vi "Main Loop.vi"(8 "error in (no error)":errorcluster, 10 "Chart Notifier":refnum<notifier>, 11 "Message Queues":T1) -> (0 "error out":errorcluster)   [LabVIEW 2018, in "Centrifuge Module.lvlib" / "Centrifuge Module Engine.lvlib"]
uses:
  Centrifuge Module Engine.lvlib
  All Message Queues.ctl
  support/Message Queue/Message Cluster.ctl
  State Cluster.ctl
  State Enum.ctl
  Centrifuge Module Settings Cluster.ctl
  EPOS4/Controls/Device Selection.ctl
  EPOS4/Controls/EPOS Communication Settings.ctl
  Centrifuge Module Display.ctl
  <vilib>/Platform/TimedLoop/XDataNode/timing_clust.ctl
  <vilib>/Platform/TimedLoop/XDataNode/nitl_modes.ctl
  <vilib>/Platform/TimedLoop/XDataNode/wakeup.ctl
  Tag VIs/Tag FGV Operation Enum.ctl
  support/Message Queue/Enqueue Message (Single).vi
  <vilib>/Platform/TimedLoop/XDataNode/XDataNode.xnode
  support/Message Queue/Message Queue.lvlib
  <vilib>/Platform/TimedLoop/XDataNode/XDNodeRunTimeDep.lvlib
  Centrifuge Module.lvlib
  Shared Variables/Dynamic Shared Variables.lvlib
  support/Support Library.lvlib
  EPOS4/EPOS4.lvlib
panel:
  out "Period (s)":dbl format="%_4g"
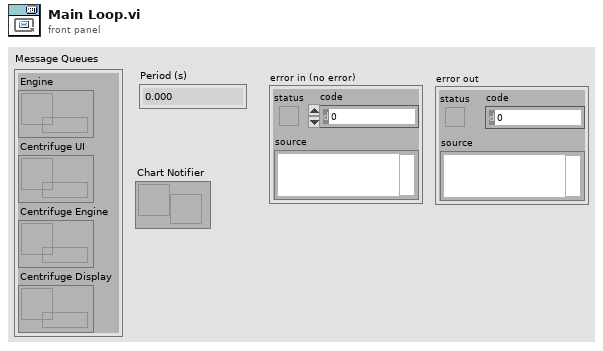
[diagram p1: front panel]
types:
  T1 = typedef "Centrifuge Module.lvlib/All Message Queues.ctl" = cluster{"Engine":refnum<queue>, "Centrifuge UI":refnum<queue>, "Centrifuge Engine":refnum<queue>, "Centrifuge Display":refnum<queue>}
  T2 = typedef "Centrifuge Module.lvlib/Centrifuge Module Display.ctl" = cluster{"Centrifuge On?":enum16{"Off", "On", "Not Initialized"}, "Cycle Period":dbl, "Current Centrifuge Speed":dbl, "Output":T3}
  T3 = typedef "Device Selection.ctl" = enum16{"Default", "EPOS4"}
  T4 = typedef "XDNodeRunTimeDep.lvlib/timing_clust.ctl" = cluster{"Expected End [f-1]":u64, "Actual End [f-1]":u64, "Finished Late? [f-1]":bool, "Expected End [i-1]":u64, "Actual End [i-1]":u64, "Finished Late? [i-1]":bool, "Expected Start [i]":u64, "Actual Start [i]":u64, "Expected Start [f]":u64, "Actual Start [f]":u64, "Source Name":string, "Structure Name":string, "Period":i64, "Deadline":i64, "Offset":i64, "Start":i64, "Priority":i32, "Timeout":i32, "Mode":T5, "Wakeup Reason":T6, "Error":errorcluster, "Source Type":string, "Secondary Source Type":string, "Global End Time":u64, "Global Start Time":u64, "Frame Duration":u64, "Iteration Duration":u64, "Assigned CPU":i32, "I/O Scan Engine Mode":u32}
  T5 = typedef "XDNodeRunTimeDep.lvlib/nitl_modes.ctl" = enum32{"No Change", "Process missed periods, maintain original phase", "Discard missed periods, maintain original phase", "Process missed periods, ignore original phase", "Discard missed periods, ignore original phase"}
  T6 = typedef "XDNodeRunTimeDep.lvlib/wakeup.ctl" = enum32{"Normal", "Aborted", "Asynchronous wakeup", "Timing source error", "Timed loop error", "Timeout"}
  T7 = cluster{"enable? (F)":bool, "name":string, "alarm on":bool, "priority":u32, "ack type":enum16{"Auto", "User", "None", "Each Occurrence"}, "area":string, "description":string, "log? (T)":bool}
  T8 = typedef "Tag FGV Operation Enum.ctl" = enum16{"Init", "Set Notification Queue", "Create Tag", "Commit", "Write Tag (Numeric)", "Write Tag (Boolean)", "Read All Tags", "Read One Tag", "Delete Tag Category", "Set Alarm Parameters (Numeric)", "Set Alarm Parameters (Boolean)", "Enable All Alarms", "Disable All Alarms", "Delete All Tags", "Read Alarms", "Ack Alarm", "Read Alarm Parameters (Numeric)", "Read Alarm Parameters (Boolean)"}
  T9 = enum32{"u32BitField", "bool", "double", "string", "int8", "uint8", "int16", "uint16", "int32", "uint32", "int64", "uint64", "single", "double waveform", "int16 waveform", "array of boolean", "array of int8", "array of uint8", "array of int16", "array of uint16", "array of int32", "array of uint32", "array of int64", "array of uint64", "array of single", "array of double", "array of double waveform", "array of int16 waveform", "array of string", "variant", "timestamp", "fixed point", "custom"}
  T10 = typedef "Centrifuge Module.lvlib/Centrifuge Module Engine.lvlib/State Enum.ctl" = enum16{"Measuring", "Idle", "Paused"}
  T11 = typedef "Centrifuge Module.lvlib/Centrifuge Module Engine.lvlib/State Cluster.ctl" = cluster{"State":T10, "Start Time":timestamp, "Configuration":T12, "Current Time":timestamp, "First Iteration":bool, "Data":cluster{"Centrifuge Speed":dbl}, "Process Name":string, "Centrifuge On?":enum16{"Off", "On", "Not Initialized"}, "Output Error":bool, "Log Started":bool}
  T12 = typedef "Centrifuge Module.lvlib/Centrifuge Module Settings Cluster.ctl" = cluster{"Cycle Period":dbl, "Manual Entry":dbl, "Output Device":T3, "EPOS4 Settings":T13}
  T13 = typedef "EPOS4.lvlib/EPOS Communication Settings.ctl" = cluster{"VISA resource name":refnum<visa-resource-name>, "axis":cluster{"keyHandle":u32, "nodeId":u16}, "Simulated?":bool}
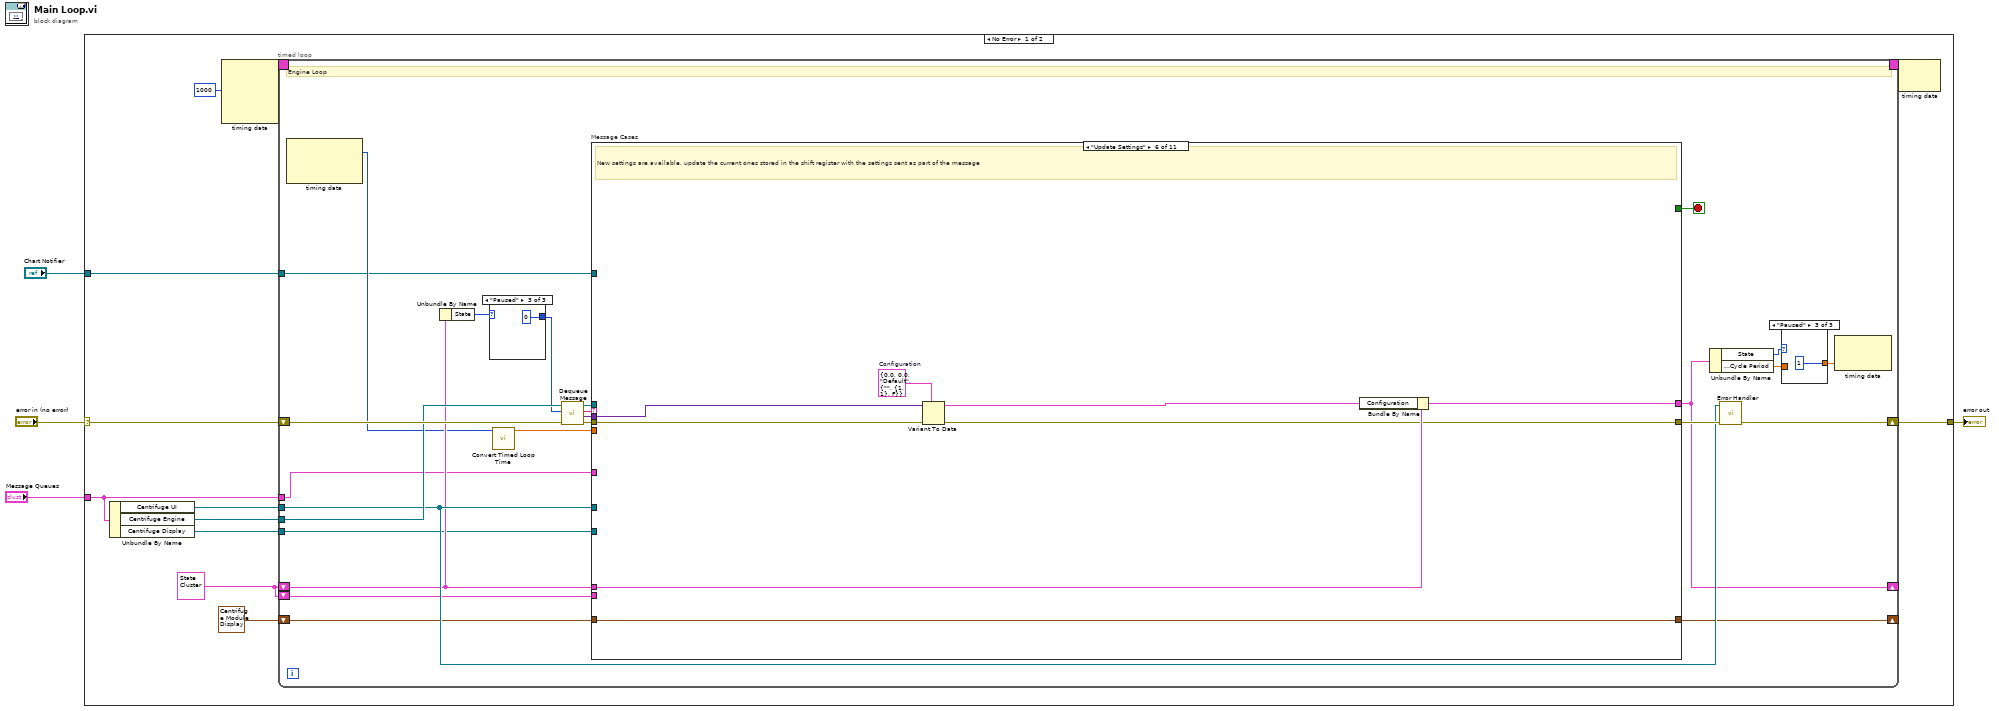
[diagram p0: block diagram]
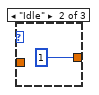
[diagram p3: hidden frame]
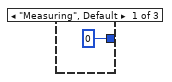
[diagram p4: hidden frame]
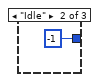
[diagram p5: hidden frame]
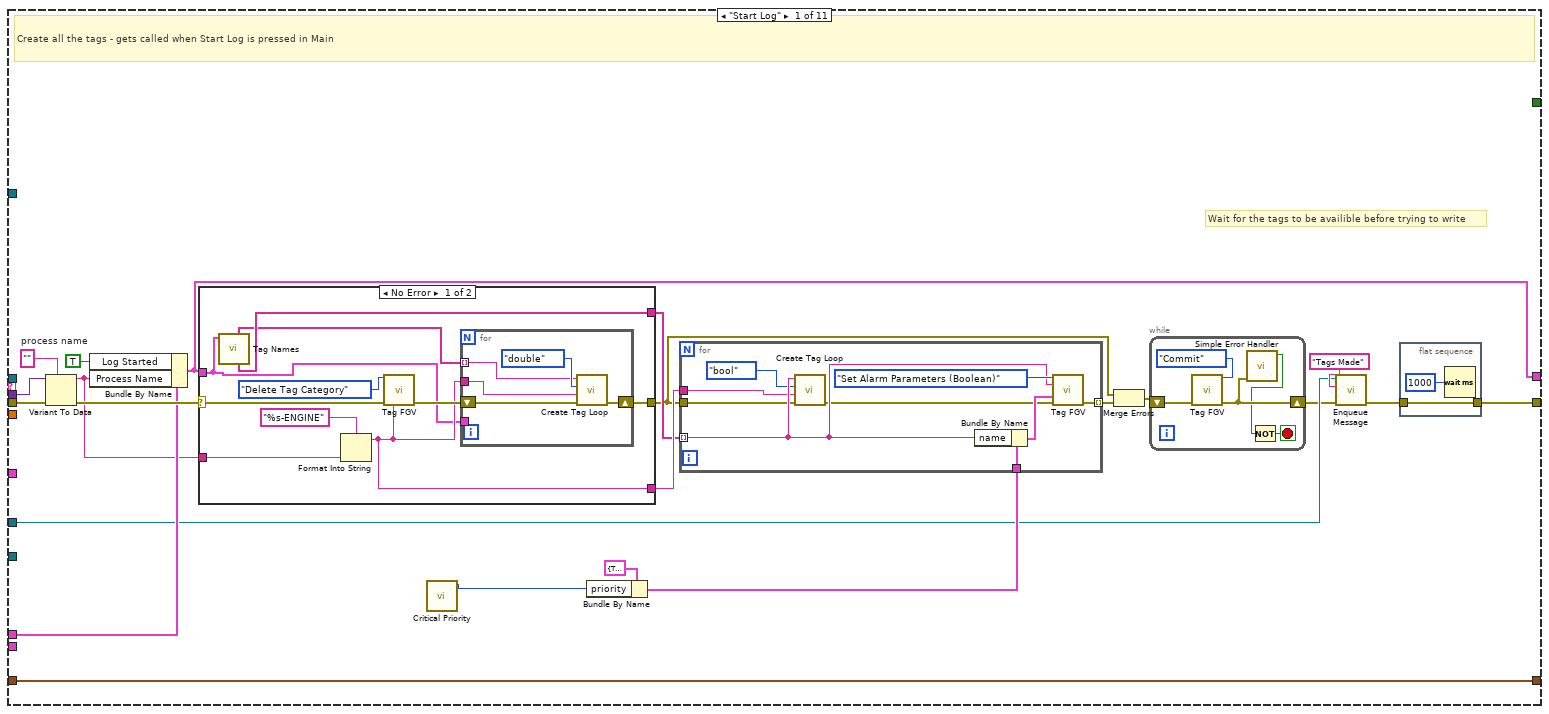
[diagram p6: hidden frame]
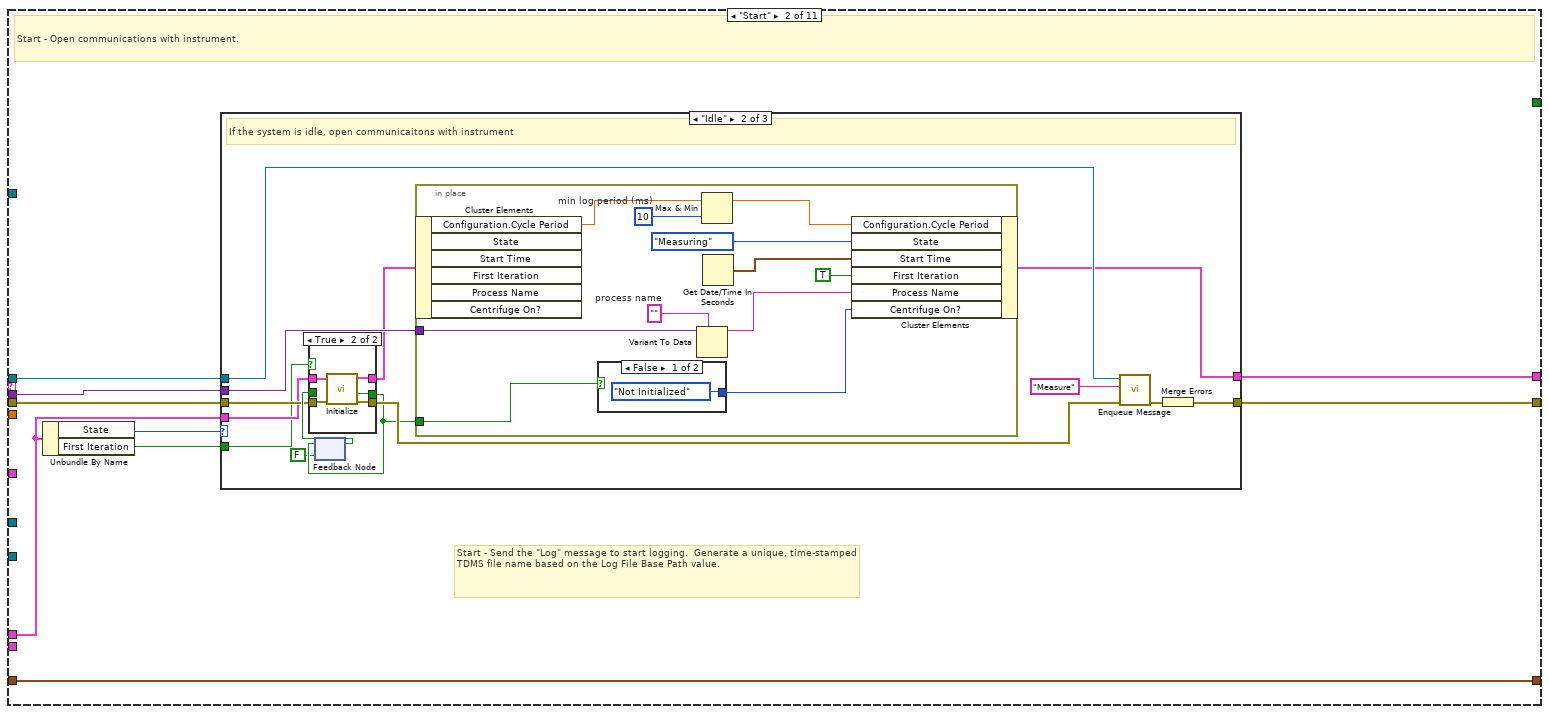
[diagram p8: hidden frame]
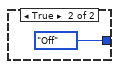
[diagram p10: hidden frame]
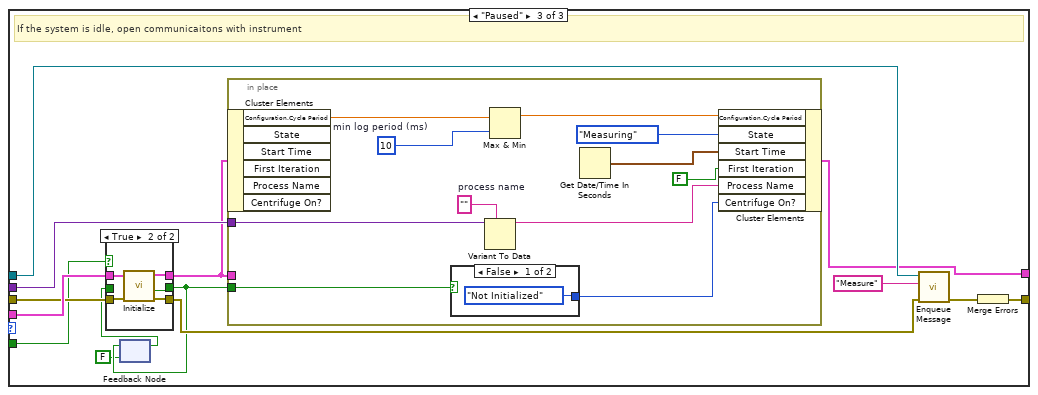
[diagram p12: hidden frame]
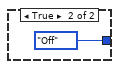
[diagram p13: hidden frame]
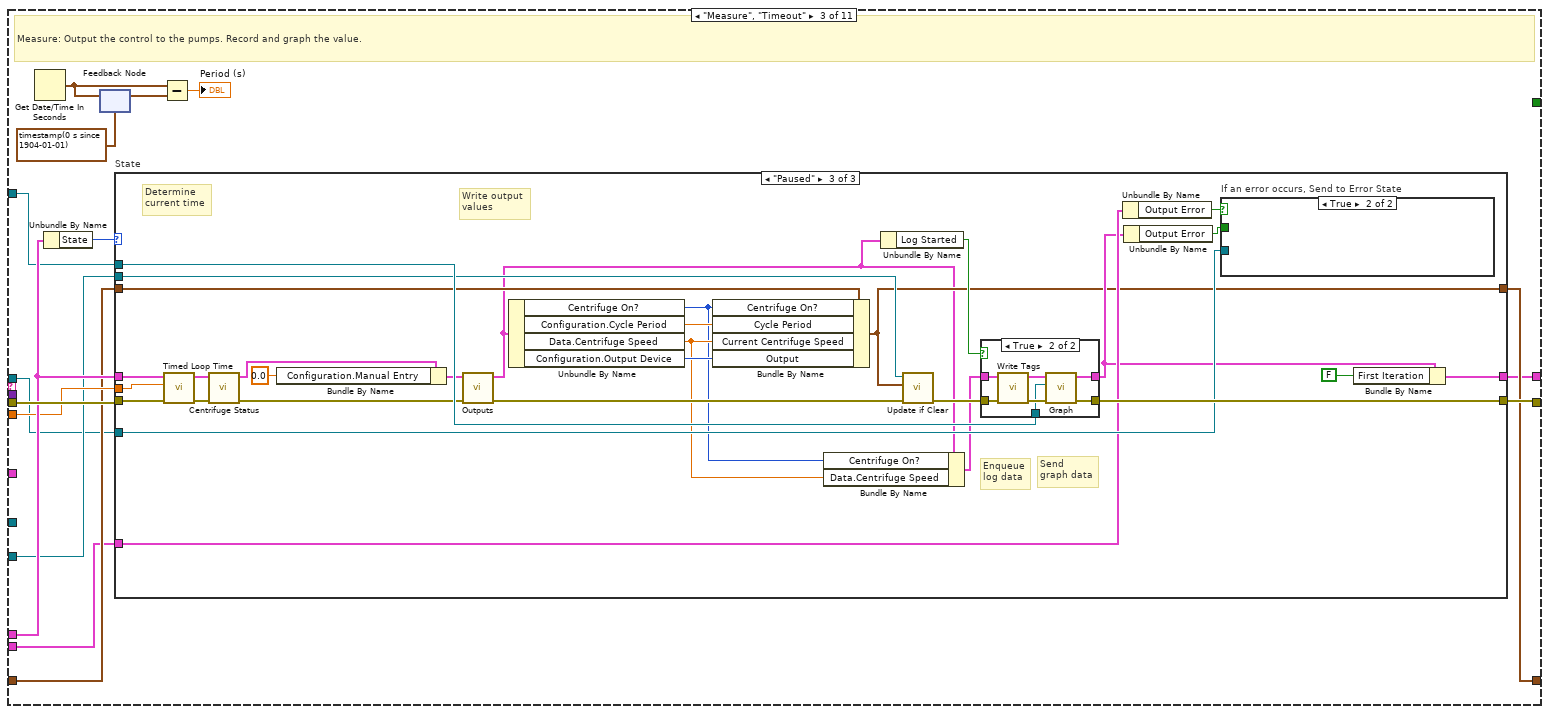
[diagram p15: hidden frame]
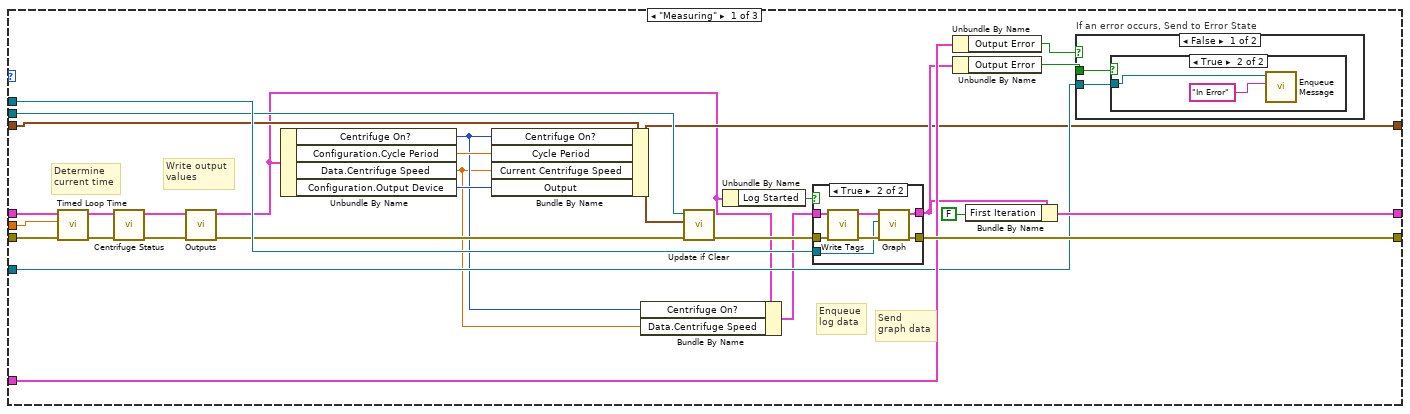
[diagram p16: hidden frame]
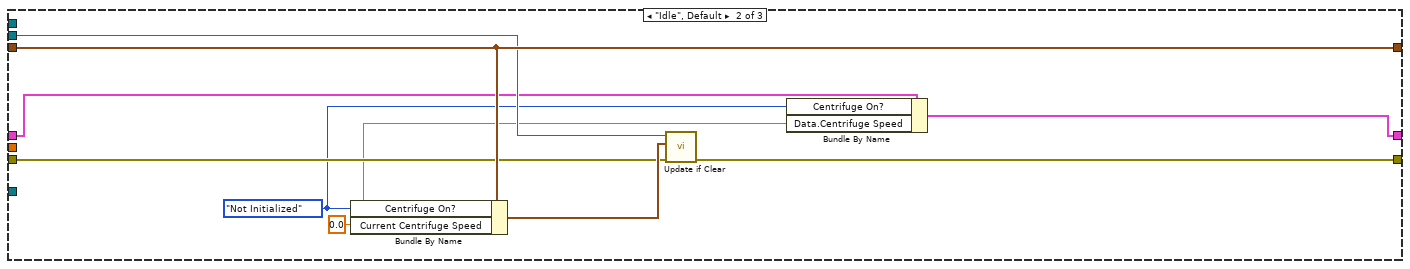
[diagram p20: hidden frame]
diagram:
  n1 = case shown="No Error" "error in (no error)" {
    selector: "error in (no error)" -> [w15 w414]
    tunnel: "Message Queues" -> [w11 _]
    tunnel: [w16 w414] -> w3
    tunnel: "Chart Notifier" -> [w9 _]
    frame No Error {
      w6 = T11 {"State"=enum."Idle", "Start Time"=timestamp(0 s since 1904-01-01), "Configuration"={"Cycle Period"=0.0, "Manual Entry"=0.0, "Output Device"=enum."Default", "EPOS4 Settings"={"VISA resource name"="", "axis"={"keyHandle"=1, "nodeId"=1}, "Simulated?"=FALSE}}, "Current Time"=timestamp(0 s since 1904-01-01), "First Iteration"=FALSE, "Data"={"Centrifuge Speed"=0.0}, "Process Name"="", "Centrifuge On?"=enum."Off", "Output Error"=FALSE, "Log Started"=FALSE}
      n2 = Unbundle By Name(w11) -> ("Centrifuge UI"=w14:refnum<queue>, "Centrifuge Engine"=w10:refnum<queue>, "Centrifuge Display"=w8:refnum<queue>)
      n3 = node-c288(i64 1000 ("Period")) -> (w13:T4)  [unwired: 3 in]
      n4 = timed-loop {
        tunnel: w10 -> [w35]
        shift-right: [w17] -> _
        shift-left: w6 -> [w31]
        shift-right: [w33] -> w16
        shift-left: w15 -> [w40]
        tunnel: w14 -> [w32]
        timing: w13 -> [_]
        timing-out: [_] -> w12
        tunnel: w11 -> [w23]
        tunnel: w9 -> [w22]
        tunnel: w8 -> [w21]
        shift-right: [w20] -> _
        shift-left: T2 {"Centrifuge On?"=enum."Off", "Cycle Period"=500.0, "Current Centrifuge Speed"=0.0, "Output"=enum."Default"} ("PM Display") -> [w19]
        shift-left: w6 -> [w18]
        stop <- w41 stop-if-true
        # "Engine Loop"
        n5 = node-c288() -> (w25:i64)  [unwired: 1 in, 2 out]
        n6 = Unbundle By Name(w31) -> ("State"=w30:T10)
        n7 = case shown="\"Paused\"" w30 {
          tunnel: [0 ("timeout in ms (-1)") -1 ("timeout in ms (-1)") 0 ("timeout in ms (-1)")] -> w29
          frame "Measuring", Default {
          }
          frame "Idle" {
          }
          frame "Paused" {
          }
        }
        n8 = call "Convert Timed Loop Time.vi"("Actual Start [i]"=w25) -> ("ET since start (s)"=w24:dbl)  [unwired: 10 in]
        n9 = call "Dequeue Message.vi"("error in (no error)"=w40, "timeout in ms (-1)"=w29, "Message Queue"=w35) -> ("error out"=w39:errorcluster, "Message Data"=w37:variant, "Message"=w38:string, "dup Message Queue"=w36:refnum<queue>)  [unwired: 5 in]
        n10 = case "Message Cases" shown="\"Update Settings\"" w38 {
          selector: w38 -> [_ _ _ _ _ _ _ _ _ _ w403]
          tunnel: w36 -> [_ w114 w191 _ _ _ w357 _ w373 _ _]
          tunnel: w39 -> [w58 w113 w201 w302 w328 w351 w360 w367 w383 w401 _]
          tunnel: [w54 w115 w202 w297 w324 w347 w362 w366 w378 w400 w402] -> w34
          tunnel: w31 -> [w64 w110 w200 w304 w329 w348 w353 w364 w382 w398 w408]
          tunnel: [w60 w107 w189 w303 w331 w346 w353 w364 w379 w396 w408] -> w17
          tunnel: [_ _ _ _ _ _ TRUE _ _ _ _] -> w41
          tunnel: w37 -> [w73 w111 _ _ _ w352 _ _ _ _ _]
          tunnel: w32 -> [w61 _ _ w306 _ _ w361 _ _ _ _]
          tunnel: w24 -> [_ _ w199 _ _ _ _ _ _ _ _]
          tunnel: w23 -> [_ _ _ _ _ _ _ _ _ _ _]
          tunnel: w22 -> [_ _ w195 _ _ _ _ _ _ _ _]
          tunnel: w21 -> [_ _ w194 w300 w326 _ _ _ w372 _ _]
          tunnel: w19 -> [w74 w109 w193 w299 w325 w349 w354 w365 w376 w399 w409]
          tunnel: [w74 w109 w192 w299 w325 w349 w354 w365 w371 w399 w409] -> w20
          tunnel: w18 -> [_ _ w190 _ _ _ _ _ _ _ _]
          frame "Start Log" {
            w72 = ""  # process name
            # "Wait for the tags to be availible before trying to write"
            # "Create all the tags - gets called when Start Log is pressed in Main"
            n11 = Variant To Data(error in=w58, type=w72, Variant=w73) -> (data=w59:string, error out=w71:errorcluster)
            n12 = Bundle By Name(cluster=w64, "Log Started"=TRUE, "Process Name"=w59) -> (w60:T11)
            n13 = case shown="No Error" w71 {
              selector: w71 -> [w97 w106]
              tunnel: [w100 w106] -> w53
              tunnel: [w95 _] -> w67
              tunnel: [w94 _] -> w66
              tunnel: w60 -> [w91 _]
              tunnel: w59 -> [w93 _]
              frame No Error {
                n14 = call "Tag Names.vi"("State In"=w91) -> ("All Boolean Tags"=w94:string[], "All  Numeric Tags"=w92:string[])  [unwired: 8 in, 1 out]
                n15 = Format Into String(format string="%s-ENGINE", w93) -> (resulting string=w95:string)  [unwired: 2 in, 1 out]
                n16 = call "Tag FGV.vi"("Operation"=Tag_FGV_Operation_Enum."Delete Tag Category", "error in (no error)"=w97, "Tag Category"=w95) -> ("error out"=w96:errorcluster)  [unwired: 5 in, 7 out]
                n17 = for {
                  shift-right: [w101] -> w100
                  shift-left: w96 -> [w102]
                  tunnel: w95 -> [w103]
                  tunnel: w92 -> [w104] mode=indexing
                  tunnel: w91 -> [_]
                  n18 = call "Create Tag Loop.vi"("error in (no error)"=w102, "Tag Category"=w103, "data type"=T9."double", "Tag Name"=w104) -> ("error out"=w101:errorcluster)  [unwired: 7 in]
                }
              }
              frame Error {
              }
            }
            n19 = call "Critical Priority.vi"() -> ("critical priority"=w70:i32)  [unwired: 11 in]
            n20 = Bundle By Name(cluster=T7 {"enable? (F)"=TRUE, "name"="Boolean", "alarm on"=TRUE, "priority"=1, "ack type"=enum."Each Occurrence", "area"="a", "description"="", "log? (T)"=TRUE} ("Boolean alarm settings"), "priority"=w70) -> (w68:T7)
            n21 = for {
              tunnel: w68 -> [w90]
              tunnel: [w89] -> w65 mode=indexing
              tunnel: w66 -> [w86] mode=indexing
              tunnel: w53 -> [w83]
              tunnel: w67 -> [w84]
              n22 = call "Create Tag Loop.vi"("error in (no error)"=w83, "Tag Category"=w84, "data type"=T9."bool", "Tag Name"=w86) -> ("error out"=w82:errorcluster)  [unwired: 7 in]
              n23 = Bundle By Name(cluster=w90, "name"=w86) -> (w88:T7)
              n24 = call "Tag FGV.vi"("Operation"=Tag_FGV_Operation_Enum."Set Alarm Parameters (Boolean)", "Tag Name"=w86, "Data"=w88, "error in (no error)"=w82) -> ("error out"=w89:errorcluster)  [unwired: 4 in, 7 out]
            }
            n25 = Merge Errors(w53, w65) -> (w57:errorcluster)
            n26 = while {
              shift-right: [w79] -> w56
              shift-left: w57 -> [w80]
              stop <- w77 stop-if-true
              n27 = call "Tag FGV.vi"("Operation"=Tag_FGV_Operation_Enum."Commit", "error in (no error)"=w80) -> ("error out"=w79:errorcluster)  [unwired: 6 in, 7 out]
              n28 = call <vilib>:"Simple Error Handler.vi"("error in (no error)"=w79) -> ("error?"=w78:bool)  [unwired: 4 in, 4 out]
              n29 = Not(x=w78) -> (.not. x?=w77:bool)
            }
            n30 = call-poly "Enqueue Message.vi"("error in (no error)"=w56, "Message"="Tags Made", "Message Queue"=w61) -> ("error out"=w55:errorcluster)  [unwired: 7 in, 1 out]
            n31 = flat-sequence {
              tunnel: [w75] -> w54
              tunnel: w55 -> [w75]
              frame #0 {
                n32 = Wait (ms)(milliseconds to wait=u32 1000) -> ()  [unwired: 1 out]
              }
            }
          }
          frame "Start" {
            # "Start - Send the \"Log\" message to start logging.  Generate a unique, time-stamped TDMS file name based on the Log File Base Path value."
            # "Start - Open communications with instrument."
            n33 = Unbundle By Name(w110) -> ("State"=w112:T10, "First Iteration"=w108:bool)
            n34 = case shown="\"Idle\"" w112 {
              tunnel: [w116 w131 w166] -> w115
              tunnel: w114 -> [_ w128 w163]
              tunnel: w113 -> [w116 w125 w160]
              tunnel: w110 -> [w117 w124 w161]
              tunnel: [w117 w119 w154] -> w107
              tunnel: w111 -> [_ w127 w162]
              tunnel: w108 -> [_ w121 w156]
              frame "Measuring", Default {
                # "The system is already running. Ignore the \"Start\" message."
              }
              frame "Idle" {
                # "If the system is idle, open communicaitons with instrument"
                n35 = feedback #1(FALSE ("Initialized")) -> (w126:bool)
                n36 = case shown="True" w121 {
                  tunnel: w125 -> [w146 w151]
                  tunnel: w124 -> [w147 w152]
                  tunnel: [w147 w150] -> w120
                  tunnel: [w146 w148] -> w123
                  tunnel: [w145 w149] -> w122
                  tunnel: w126 -> [w145 _]
                  frame False {
                  }
                  frame True {
                    n37 = call "Initialize.vi"("error in (no error)"=w151, "State in"=w152) -> ("error out"=w148:errorcluster, "Initialized"=w149:bool, "State out"=w150:T11)  [unwired: 7 in]
                  }
                }
                n38 = feedback-in #1(w122) -> ()
                n39 = in-place {
                  in-place-border: w127 -> [w140]
                  in-place-border: w122 -> [w139]
                  w141 = ""  # process name
                  w142 = 10  # min log period (ms)
                  n40 = in-place-cluster #2(w120) -> ("Configuration.Cycle Period"=w138:dbl)  [unwired: 5 out]
                  n41 = case shown="False" w139 {
                    tunnel: [enum16{"Off", "On", "Not Initialized"}."Not Initialized" ("Pump On?") enum16{"Off", "On", "Not Initialized"}."Off" ("Pump On?")] -> w132
                    frame False {
                    }
                    frame True {
                    }
                  }
                  n42 = Variant To Data(type=w141, Variant=w140) -> (data=w133:string)  [unwired: 1 in, 1 out]
                  n43 = Max & Min(x=w138, y=w142) -> (max(x,y)=w137:dbl)  [unwired: 1 out]
                  n44 = Get Date/Time In Seconds() -> (seconds since 1Jan1904=w135:timestamp)
                  n45 = in-place-cluster #2("Configuration.Cycle Period"=w137, "State"=State_Enum."Measuring", "Start Time"=w135, "First Iteration"=TRUE, "Process Name"=w133, "Centrifuge On?"=w132) -> (w119:T11)
                }
                n46 = call-poly "Enqueue Message.vi"("error in (no error)"=w123, "Message"="Measure", "Message Queue"=w128) -> ("error out"=w129:errorcluster)  [unwired: 7 in, 1 out]
                n47 = Merge Errors(w129) -> (w131:errorcluster)
              }
              frame "Paused" {
                # "If the system is idle, open communicaitons with instrument"
                n48 = feedback #3(FALSE ("Initialized")) -> (w157:bool)
                n49 = case shown="True" w156 {
                  tunnel: w160 -> [w181 w186]
                  tunnel: w161 -> [w182 w187]
                  tunnel: [w182 w185] -> w155
                  tunnel: [w181 w183] -> w159
                  tunnel: [w180 w184] -> w158
                  tunnel: w157 -> [w180 _]
                  frame False {
                  }
                  frame True {
                    n50 = call "Initialize.vi"("error in (no error)"=w186, "State in"=w187) -> ("error out"=w183:errorcluster, "Initialized"=w184:bool, "State out"=w185:T11)  [unwired: 7 in]
                  }
                }
                n51 = feedback-in #3(w158) -> ()
                n52 = in-place {
                  in-place-border: w162 -> [w175]
                  in-place-border: w155 -> [_]
                  in-place-border: w158 -> [w174]
                  w176 = ""  # process name
                  w177 = 10  # min log period (ms)
                  n53 = in-place-cluster #4(w155) -> ("Configuration.Cycle Period"=w173:dbl)  [unwired: 5 out]
                  n54 = case shown="False" w174 {
                    tunnel: [enum16{"Off", "On", "Not Initialized"}."Not Initialized" ("Pump On?") enum16{"Off", "On", "Not Initialized"}."Off" ("Pump On?")] -> w167
                    frame False {
                    }
                    frame True {
                    }
                  }
                  n55 = Variant To Data(type=w176, Variant=w175) -> (data=w168:string)  [unwired: 1 in, 1 out]
                  n56 = Max & Min(x=w173, y=w177) -> (max(x,y)=w172:dbl)  [unwired: 1 out]
                  n57 = Get Date/Time In Seconds() -> (seconds since 1Jan1904=w170:timestamp)
                  n58 = in-place-cluster #4("Configuration.Cycle Period"=w172, "State"=State_Enum."Measuring", "Start Time"=w170, "First Iteration"=FALSE, "Process Name"=w168, "Centrifuge On?"=w167) -> (w154:T11)
                }
                n59 = call-poly "Enqueue Message.vi"("error in (no error)"=w159, "Message"="Measure", "Message Queue"=w163) -> ("error out"=w164:errorcluster)  [unwired: 7 in, 1 out]
                n60 = Merge Errors(w164) -> (w166:errorcluster)
              }
            }
          }
          frame "Measure", "Timeout" {
            # "Measure: Output the control to the pumps. Record and graph the value."
            n61 = Get Date/Time In Seconds() -> (seconds since 1Jan1904=w197:timestamp)
            n62 = Unbundle By Name(w200) -> ("State"=w203:T10)
            n63 = feedback-in #5(w197) -> ()
            n64 = feedback #5(timestamp(0 s since 1904-01-01) ("seconds since 1Jan1904")) -> (w198:timestamp)
            n65 = case "State" shown="\"Paused\"" w203 {
              tunnel: w201 -> [w230 w250 w277]
              tunnel: w200 -> [w229 w248 w278]
              tunnel: [w231 w249 w272] -> w202
              tunnel: [w227 w245 w265] -> w189
              tunnel: w199 -> [w228 _ w282]
              tunnel: w195 -> [w225 _ w283]
              tunnel: w194 -> [w212 w252 w263]
              tunnel: w193 -> [w222 w253 w281]
              tunnel: [w211 w253 w262] -> w192
              tunnel: w191 -> [w213 _ w271]
              tunnel: w190 -> [w215 _ w269]
              frame "Measuring" {
                # "Determine\ncurrent time"
                # "Send\ngraph data"
                # "Enqueue\nlog data"
                # "Write output\nvalues"
                n66 = call "Timed Loop Time.vi"("error in (no error)"=w230, "ET since start (s)"=w228, "State in"=w229) -> ("error out"=w221:errorcluster, "State out"=w220:T11)  [unwired: 7 in]
                n67 = call "Centrifuge Status.vi"("error in (no error)"=w221, 11:w220) -> ("error out"=w223:errorcluster, "State out"=w224:T11)  [unwired: 8 in]
                n68 = call "Outputs.vi"("error in (no error)"=w223, "State in"=w224) -> ("error out"=w210:errorcluster, "State out"=w207:T11)  [unwired: 8 in]
                n69 = Unbundle By Name(w207) -> ("Centrifuge On?"=w205:enum16{"Off", "On", "Not Initialized"}, "Configuration.Cycle Period"=w219:dbl, "Data.Centrifuge Speed"=w204:dbl, "Configuration.Output Device"=w208:T3)
                n70 = Bundle By Name(cluster=w222, "Centrifuge On?"=w205, "Cycle Period"=w219, "Current Centrifuge Speed"=w204, "Output"=w208) -> (w211:T2)
                n71 = Bundle By Name(cluster=w207, "Centrifuge On?"=w205, "Data.Centrifuge Speed"=w204) -> (w206:T11)
                n72 = call "Update if Clear.vi"("error in (no error)"=w210, "Message Data"=w211, "Queue in"=w212) -> ("error out"=w209:errorcluster)  [unwired: 8 in]
                n73 = Unbundle By Name(w207) -> ("Log Started"=w218:bool)
                n74 = case shown="True" w218 {
                  tunnel: [w236 w242] -> w231
                  tunnel: [w237 w241] -> w214
                  tunnel: w225 -> [_ w240]
                  tunnel: w206 -> [w237 w239]
                  tunnel: w209 -> [w236 w238]
                  frame False {
                  }
                  frame True {
                    n75 = call "Write Tags.vi"("error in (no error)"=w238, "State in"=w239) -> ("error out"=w243:errorcluster, "State out"=w244:T11)  [unwired: 8 in]
                    n76 = call "Graph.vi"("error in (no error)"=w243, "notifier out"=w240, "State in"=w244) -> ("error out"=w242:errorcluster, "State out"=w241:T11)  [unwired: 7 in]
                  }
                }
                n77 = Unbundle By Name(w215) -> ("Output Error"=w216:bool)
                n78 = Unbundle By Name(w214) -> ("Output Error"=w217:bool)
                n79 = Bundle By Name(cluster=w214, "First Iteration"=FALSE) -> (w227:T11)
                n80 = case "If an error occurs, Send to Error State" shown="False" w216 {
                  tunnel: w217 -> [w233 _]
                  tunnel: w213 -> [w232 _]
                  frame False {
                    n81 = case shown="True" w233 {
                      tunnel: w232 -> [_ w234]
                      frame False {
                      }
                      frame True {
                        n82 = call-poly "Enqueue Message.vi"("Message"="In Error", "Message Queue"=w234) -> ()  [unwired: 8 in, 2 out]
                      }
                    }
                  }
                  frame True {
                  }
                }
              }
              frame "Idle", Default {
                w246 = 0.0 ("Current Pump Speed")
                w247 = enum16{"Off", "On", "Not Initialized"}."Not Initialized" ("Pump On?")
                n83 = Bundle By Name(cluster=w253, "Centrifuge On?"=w247, "Current Centrifuge Speed"=w246) -> (w251:T2)
                n84 = call "Update if Clear.vi"("error in (no error)"=w250, "Message Data"=w251, "Queue in"=w252) -> ("error out"=w249:errorcluster)  [unwired: 8 in]
                n85 = Bundle By Name(cluster=w248, "Centrifuge On?"=w247, "Data.Centrifuge Speed"=w246) -> (w245:T11)
              }
              frame "Paused" {
                # "Determine\ncurrent time"
                # "Write output\nvalues"
                # "Send\ngraph data"
                # "Enqueue\nlog data"
                n86 = call "Timed Loop Time.vi"("error in (no error)"=w277, "ET since start (s)"=w282, "State in"=w278) -> ("error out"=w274:errorcluster, "State out"=w276:T11)  [unwired: 7 in]
                n87 = call "Centrifuge Status.vi"("error in (no error)"=w274, 11:w276) -> ("error out"=w273:errorcluster, "State out"=w275:T11)  [unwired: 8 in]
                n88 = Bundle By Name(cluster=w275, "Configuration.Manual Entry"=0.0) -> (w279:T11)
                n89 = call "Outputs.vi"("error in (no error)"=w273, "State in"=w279) -> ("error out"=w261:errorcluster, "State out"=w257:T11)  [unwired: 8 in]
                n90 = Unbundle By Name(w257) -> ("Centrifuge On?"=w254:enum16{"Off", "On", "Not Initialized"}, "Configuration.Cycle Period"=w259:dbl, "Data.Centrifuge Speed"=w255:dbl, "Configuration.Output Device"=w258:T3)
                n91 = Bundle By Name(cluster=w281, "Centrifuge On?"=w254, "Cycle Period"=w259, "Current Centrifuge Speed"=w255, "Output"=w258) -> (w262:T2)
                n92 = Bundle By Name(cluster=w257, "Centrifuge On?"=w254, "Data.Centrifuge Speed"=w255) -> (w256:T11)
                n93 = Unbundle By Name(w257) -> ("Log Started"=w264:bool)
                n94 = call "Update if Clear.vi"("error in (no error)"=w261, "Message Data"=w262, "Queue in"=w263) -> ("error out"=w260:errorcluster)  [unwired: 8 in]
                n95 = case shown="False" w264 {
                  tunnel: w283 -> [_ w290]
                  tunnel: w260 -> [w284 w289]
                  tunnel: [w284 w288] -> w272
                  tunnel: w256 -> [w285 w287]
                  tunnel: [w285 w286] -> w266
                  frame False {
                  }
                  frame True {
                    n96 = call "Write Tags.vi"("error in (no error)"=w289, "State in"=w287) -> ("error out"=w292:errorcluster, "State out"=w291:T11)  [unwired: 8 in]
                    n97 = call "Graph.vi"("error in (no error)"=w292, "notifier out"=w290, "State in"=w291) -> ("error out"=w288:errorcluster, "State out"=w286:T11)  [unwired: 7 in]
                  }
                }
                n98 = Unbundle By Name(w269) -> ("Output Error"=w268:bool)
                n99 = Unbundle By Name(w266) -> ("Output Error"=w270:bool)
                n100 = case "If an error occurs, Send to Error State" shown="True" w268 {
                  tunnel: w270 -> [w294 _]
                  tunnel: w271 -> [w293 _]
                  frame False {
                    n101 = case shown="True" w294 {
                      tunnel: w293 -> [_ w296]
                      frame False {
                      }
                      frame True {
                        n102 = call-poly "Enqueue Message.vi"("Message"="In Error", "Message Queue"=w296) -> ()  [unwired: 8 in, 2 out]
                      }
                    }
                  }
                  frame True {
                  }
                }
                n103 = Bundle By Name(cluster=w266, "First Iteration"=FALSE) -> (w265:T11)
              }
            }
            n104 = Subtract(x=w197, y=w198) -> (x-y=→"Period (s)":dbl)
          }
          frame "Stop" {
            # "Stop - Flush the message queue of any pending \"Log\" messages. Call 'Flush Data to Log File.vi' so any pending data is not lost."
            n105 = call <vilib>:"Clear Errors.vi"("error in (no error)"=w302) -> ("error out"=w301:errorcluster)  [unwired: 5 in, 1 out]
            n106 = Unbundle By Name(w304) -> ("State"=w305:T10)
            n107 = case shown="\"Measuring\", Default" w305 {
              tunnel: [w311 w317] -> w298
              tunnel: w301 -> [w308 w317]
              tunnel: w306 -> [w315 _]
              tunnel: w304 -> [w309 w316]
              tunnel: [w313 w316] -> w303
              frame "Measuring", Default {
                # "If the system is logging, stop logging."
                n108 = call "Close.vi"("error in (no error)"=w308, "State in"=w309) -> ("error out"=w307:errorcluster, "State out"=w310:T11)  [unwired: 7 in, 1 out]
                n109 = Bundle By Name(cluster=w310, "State"=State_Enum."Idle") -> (w313:T11)
                n110 = call-poly "Enqueue Message.vi"("error in (no error)"=w307, "Message"="Logging Stopped", "Message Queue"=w315) -> ("error out"=w311:errorcluster)  [unwired: 7 in, 1 out]
              }
              frame "Idle" {
                # "The system is already idle. Ignore the \"Stop\" message."
              }
            }
            n111 = call "Update if Clear.vi"("error in (no error)"=w298, "Message Data"=w299, "Queue in"=w300) -> ("error out"=w297:errorcluster)  [unwired: 8 in]
          }
          frame "Pause" {
            # "Stop - Flush the message queue of any pending \"Log\" messages. Call 'Flush Data to Log File.vi' so any pending data is not lost."
            n112 = Unbundle By Name(w329) -> ("First Iteration"=w330:bool)
            n113 = case shown="True" w330 {
              tunnel: w329 -> [w332 w337]
              tunnel: [w332 w341] -> w327
              tunnel: w328 -> [w333 w338]
              tunnel: [w333 w339] -> w320
              frame False {
              }
              frame True {
                # "If we start on a pause condition, initialize the pump"
                n114 = call "Initialize.vi"("error in (no error)"=w338, "State in"=w337) -> ("error out"=w339:errorcluster, "Initialized"=w340:bool, "State out"=w336:T11)  [unwired: 7 in]
                n115 = case shown="True" w340 {
                  tunnel: [enum16{"Off", "On", "Not Initialized"}."Not Initialized" ("Pump On?") enum16{"Off", "On", "Not Initialized"}."Off" ("Pump On?")] -> w334
                  tunnel: [_ FALSE] -> w335
                  frame False {
                  }
                  frame True {
                  }
                }
                n116 = Bundle By Name(cluster=w336, "Centrifuge On?"=w334, "First Iteration"=w335) -> (w341:T11)
              }
            }
            n117 = call <vilib>:"Clear Errors.vi"("error in (no error)"=w320) -> ("error out"=w321:errorcluster)  [unwired: 5 in, 1 out]
            n118 = call "Pause.vi"("error in (no error)"=w321, "State in"=w327) -> ("error out"=w319:errorcluster, "State out"=w322:T11)  [unwired: 8 in]
            n119 = Bundle By Name(cluster=w322, "State"=State_Enum."Paused") -> (w331:T11)
            n120 = Merge Errors(w319, w320) -> (w318:errorcluster)
            n121 = call "Update if Clear.vi"("error in (no error)"=w318, "Message Data"=w325, "Queue in"=w326) -> ("error out"=w324:errorcluster)  [unwired: 8 in]
          }
          frame "Update Settings" {
            w350 = T12 {"Cycle Period"=0.0, "Manual Entry"=0.0, "Output Device"=enum."Default", "EPOS4 Settings"={"VISA resource name"="", "axis"={"keyHandle"=1, "nodeId"=1}, "Simulated?"=FALSE}}  # Configuration
            # "New settings are available, update the current ones stored in the shift register with the settings sent as part of the message"
            n122 = Variant To Data(error in=w351, type=w350, Variant=w352) -> (data=w345:T12, error out=w347:errorcluster)
            n123 = Bundle By Name(cluster=w348, "Configuration"=w345) -> (w346:T11)
          }
          frame "Exit" {
            # "Release the Logging queue reference"
            # "Don't check the error out. The UI message queue may have already been released."
            # "Stop the VI"
            # "Exit - Send the Exit message to the UI Message Handler.  Call 'Flush Data to Log File.vi' so any pending data is not lost."
            n124 = Release Queue(queue=w357, error in (no error)=w360) -> (error out=w356:errorcluster)  [unwired: 1 in, 2 out]
            n125 = call-poly "Enqueue Message.vi"("Priority Message? (F)"=TRUE, "Message"="Exit", "Message Queue"=w361) -> ("error out"=w355:errorcluster)  [unwired: 7 in, 1 out]
            n126 = call <vilib>:"Clear Errors.vi"("error in (no error)"=w355) -> ()  [unwired: 5 in, 2 out]
            n127 = Merge Errors(w356) -> (w362:errorcluster)
          }
          frame "---Copy This Frame---" {
            # "Duplicate this frame when creating new messages.  Change this comment in the duplicated frame to describe this message."
            n128 = Merge Errors(w367) -> (w366:errorcluster)
          }
          frame "In Error" {
            # "If we have a disconnect Error we will go to this state, and attempt to reconnect and get back to the pre-error state"
            n129 = Merge Errors(w383) -> (w380:errorcluster)
            n130 = call "Initialize.vi"("error in (no error)"=w380, "State in"=w382) -> ("error out"=w370:errorcluster, "Initialized"=w381:bool, "State out"=w377:T11)  [unwired: 7 in]
            n131 = Unbundle By Name(w377) -> ("Data.Centrifuge Speed"=w374:dbl, "Configuration.Cycle Period"=w375:dbl, "Configuration.Output Device"=w368:T3)
            n132 = Bundle By Name(cluster=w376, "Current Centrifuge Speed"=w374, "Cycle Period"=w375, "Output"=w368) -> (w371:T2)
            n133 = call "Update if Clear.vi"("error in (no error)"=w370, "Message Data"=w371, "Queue in"=w372) -> ("error out"=w369:errorcluster)  [unwired: 8 in]
            n134 = case shown="False" w381 {
              tunnel: w373 -> [w388 w392]
              tunnel: w369 -> [w387 w391]
              tunnel: [w385 w394] -> w379
              tunnel: w377 -> [w385 w394]
              tunnel: [w384 w390] -> w378
              frame False {
                n135 = Wait (ms)(milliseconds to wait=u32 5000) -> ()  [unwired: 1 out]
                n136 = call-poly "Enqueue Message.vi"("error in (no error)"=w387, "Message"="In Error", "Message Queue"=w388) -> ("error out"=w384:errorcluster)  [unwired: 7 in, 1 out]
              }
              frame True {
                n137 = call-poly "Enqueue Message.vi"("error in (no error)"=w391, "Message"="Measure", "Message Queue"=w392) -> ("error out"=w390:errorcluster)  [unwired: 7 in, 1 out]
              }
            }
          }
          frame "Initialize" {
            # "Duplicate this frame when creating new messages.  Change this comment in the duplicated frame to describe this message."
            n138 = Merge Errors(w401) -> (w400:errorcluster)
            n139 = Bundle By Name(cluster=w398, "Log Started"=FALSE, "First Iteration"=TRUE) -> (w396:T11)
          }
          frame Default {
            # "'Default' case only runs if there is a message that isn't defined in any of the other cases.  Output a programming error."
            n140 = Concatenate Strings("The invalid message string " ("string"), w403, " was received in the Pump Module Engine." ("string")) -> (w404:string)
            n141 = Bundle By Name(cluster=errorcluster {"status"=TRUE, "code"=1, "source"=""} ("error constant"), "source"=w404) -> (w402:errorcluster)
          }
        }
        n142 = Unbundle By Name(w17) -> ("State"=w28:T10, "Configuration.Cycle Period"=w26:dbl)
        n143 = call "Error Handler.vi"("error in (no error)"=w34, "Message Queue"=w32) -> ("dup error in"=w33:errorcluster)  [unwired: 8 in, 1 out]
        n144 = case shown="\"Paused\"" w28 {
          tunnel: [w42 1 1] -> w27
          tunnel: w26 -> [w42 _ _]
          frame "Measuring" {
          }
          frame "Idle" {
          }
          frame "Paused" {
          }
        }
        n145 = node-c288(w27) -> ()  [unwired: 1 in, 1 out]
      }
      n146 = node-c288(w12) -> ()  [unwired: 1 out]
    }
    frame Error {
    }
  }
  "error out" <- w3
